vi "get_valve_position.vi"(9 "NUMBER OF VALVES":u32, 10 "CURRENT VALVE":u32) -> (0 "LAST VALVE?":bool, 2 "VALVE INDEX":u32, 3 "CURRENT VALVE":u32)   [LabVIEW 2013]
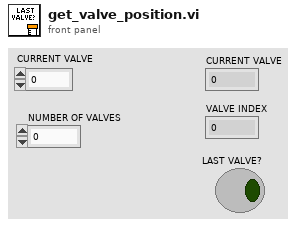
[diagram p1: front panel]
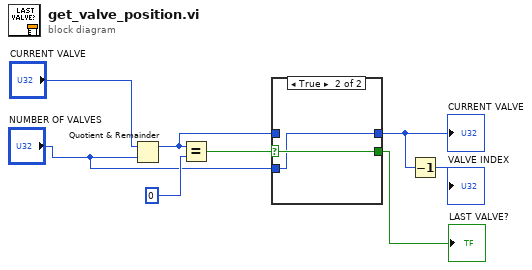
[diagram p0: block diagram]
diagram:
  n1 = Quotient & Remainder(x="CURRENT VALVE", y="NUMBER OF VALVES") -> (x-y*floor(x/y)=w6:u32)  [unwired: 1 out]
  n2 = Equal?(x=w6, y=u32 0) -> (x = y?=w5:bool)
  n3 = case shown="True" w5 {
    selector: w5 -> [w9 w12]
    tunnel: w6 -> [w10 _]
    tunnel: [w10 w11] -> w2
    tunnel: [w9 w12] -> w4
    tunnel: "NUMBER OF VALVES" -> [_ w11]
    frame False {
    }
    frame True {
    }
  }
  "LAST VALVE?" <- w4
  "CURRENT VALVE" <- w2
  n4 = Decrement(x=w2) -> (x-1=→"VALVE INDEX":u32)
